vi "ADIS16470 SPI IMU.vi"() -> ()   [LabVIEW 2025]
doc: "XRS450 SPI Gyro Example\n\nThis example shows how to use the Analog Devices XRS450 gyro connected to the SPI port on the RoboRIO.\n\nThis example expects a USB cable connected from your development PC to the Type B USB Jack (next to the power input) on the roboRIO.\n\nThis example expects the Driver Station to be running."
panel:
  out "IMU Chart":T1(graph)
  in  "Calibration (sec)":dbl=4.0
  in  "Recalibrate?":bool
  out "Calibrated?":bool
  in  "Reset?":bool
  out "Device Found":bool
  in  "stop":bool
  # "Use this example to identify the X, Y, and Z axis of\nthe IMU. It also demonstrates how reset and\nrecalibration differ and lets you explore how the length\nof calibration impacts the stability of the IMU."
  # "This shows wiring for the Analog Devices ADIS16470 IMU.  It should be plugged directly into the SPI port."
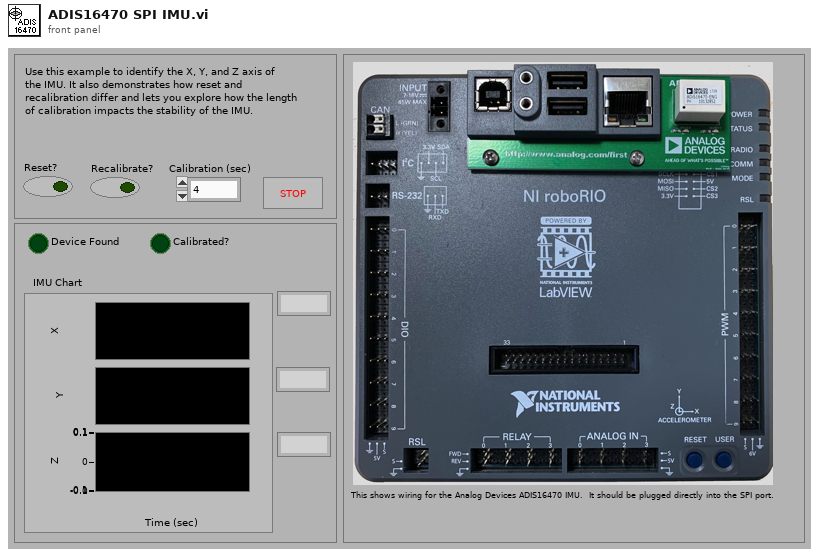
[diagram p1: front panel]
types:
  T1 = cluster{"XAngle":dbl, "YAngle":dbl, "ZAngle":dbl}
  T2 = typedef "ADIS16470 Device Reference.ctl" = cluster{"DevStatus":errorcluster, "Hardware Config":T3, "Calibration Complete":refnum<notifier>, "Status Reference":refnum<data-value>, "Data Reference":refnum<data-value>, "Sychronous Process VI":T7, "Cmd FIFO":refnum<k33>, "Source":T8, "Data FIFO":refnum<k33>, "Calibration Time (ms)":u32, "Data Reference":refnum<data-value>}
  T3 = typedef "ADIS16470 Hardware Configuration.ctl" = cluster{"SPI Clock Rate (Hz)":dbl, "IMU SPI Mode (3)":T4, "IMU Reset Pin":T5, "IMU SPI Bus":T6, "IMU Data Ready Pin":T5, "Stall Config":cluster{"Pow2BytesPerRead":u8, "StallTicks":u16, "CsToSclkTicks":u8}}
  T4 = typedef "WPI_SPIMode.ctl" = enum16{"Mode 0 (Clk Idle Low,Sample on Leading)", "Mode 1 (Clk Idle Low,Sample on Trailing)", "Mode 2 (Clk Idle High,Sample on Leading)", "Mode 3 (Clk Idle High,Sample on Trailing)"}
  T5 = typedef "FPGA_DIOChannel.ctl" = enum8{"DIO 0", "DIO 1", "DIO 2", "DIO 3", "DIO 4", "DIO 5", "DIO 6", "DIO 7", "DIO 8", "DIO 9", "DIO MXP 0", "DIO MXP 1", "DIO MXP 2", "DIO MXP 3", "DIO MXP 4", "DIO MXP 5", "DIO MXP 6", "DIO MXP 7", "DIO MXP 8", "DIO MXP 9", "DIO MXP 10", "DIO MXP 11", "DIO MXP 12", "DIO MXP 13", "DIO MXP 14", "DIO MXP 15", "SPI Port CS1", "SPI Port CS2", "SPI Port CS3", "SPI Port MISO", "SPI Port MOSI", "Invalid"}
  T6 = typedef "spi_bus.ctl" = enum16{"SPI On-Board, CS0", "SPI On-Board, CS1", "SPI On-Board, CS2", "SPI On-Board, CS3", "SPI MXP", "Invalid"}
  T7 = typedef "ADIS16470 Process.ctl" = refnum<vi>
  T8 = typedef "FPGA_CounterEncoderSourceConvertionLVSourceType.ctl" = cluster{"DevStatus":errorcluster, "AnalogTriggerMode?":bool, "DigitalMode":cluster{"DIO Channel":T9}, "AnalogTriggerMode":cluster{"AnalogTriggerIndex":T10, "OutputType":T11}}
  T9 = typedef "FPGA_DIODigitalSourceChannel.ctl" = enum8{"DIO 0", "DIO 1", "DIO 2", "DIO 3", "DIO 4", "DIO 5", "DIO 6", "DIO 7", "DIO 8", "DIO 9", "DIO MXP 0", "DIO MXP 1", "DIO MXP 2", "DIO MXP 3", "DIO MXP 4", "DIO MXP 5", "DIO MXP 6", "DIO MXP 7", "DIO MXP 8", "DIO MXP 9", "DIO MXP 10", "DIO MXP 11", "DIO MXP 12", "DIO MXP 13", "DIO MXP 14", "DIO MXP 15", "SPI Port CS1", "SPI Port CS2", "SPI Port CS3", "SPI Port MISO", "SPI Port MOSI", "Disabled"}
  T10 = typedef "FPGA_AnalogTriggerIndex.ctl" = enum8{"Trig 0", "Trig 1", "Trig 2", "Trig 3", "Trig 4", "Trig 5", "Trig 6", "Trig 7", "Invalid"}
  T11 = typedef "FPGA_AnalogTriggerOutType.ctl" = enum16{"InWindow", "TriggerState", "Rising", "Falling"}
  T12 = typedef "ADIS16470 Status.ctl" = cluster{"Calibrated?":bool, "IMU Detected?":bool}
  T13 = typedef "ADIS16470 Data.ctl" = cluster{"XAngle":dbl, "YAngle":dbl, "ZAngle":dbl}
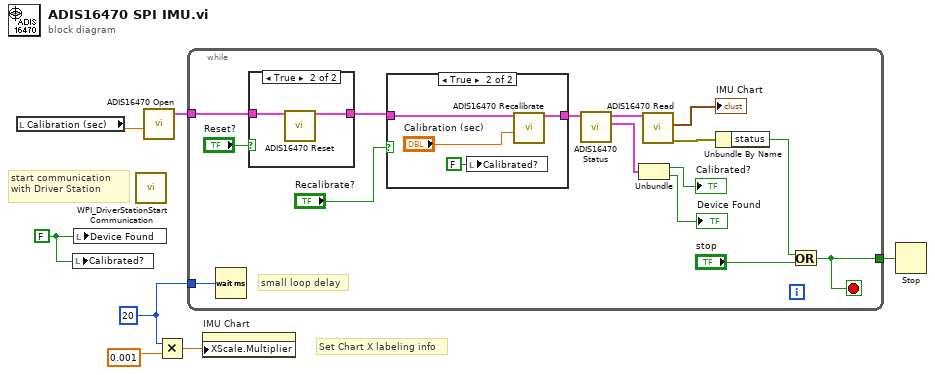
[diagram p0: block diagram]
diagram:
  w5 = u32 20 ("milliseconds to wait")
  w7 = FALSE ("Device Found")
  # "Set Chart X labeling info"
  # "start communication with Driver Station"
  n1 = local read "Calibration (sec)"() -> (w2:dbl)
  n2 = local write "Calibrated?"(w7) -> ()
  n3 = local write "Device Found"(w7) -> ()
  n4 = call <vilib>:"WPI_DriverStationStart Communication.vi"() -> ()  [unwired: 12 in]
  n5 = call <vilib>:"ADIS16470 Open.vi"("Initial Calibration Time (4s)"=w2) -> ("ADIS16470DevRef"=w1:T2)  [unwired: 9 in, 1 out]
  n6 = Multiply(x=w5, y=0.001 ("milliseconds to wait")) -> (x*y=w3:dbl)
  n7 = while {
    tunnel: w1 -> [w21]
    tunnel: [w14] -> w6
    tunnel: w5 -> [w13]
    stop <- w14 stop-if-true
    # "small loop delay"
    n8 = Wait (ms)(milliseconds to wait=w13) -> ()  [unwired: 1 out]
    n9 = case shown="True" "Reset?" {
      tunnel: w21 -> [w28 w30]
      tunnel: [w28 w29] -> w16
      frame False {
      }
      frame True {
        n10 = call <vilib>:"ADIS16470 Reset.vi"("ADIS16470DevRef"=w30) -> ("ADIS16470DevRef"=w29:T2)  [unwired: 9 in, 1 out]
      }
    }
    n11 = case shown="True" "Recalibrate?" {
      tunnel: w16 -> [w23 w26]
      tunnel: [w23 w25] -> w12
      frame False {
      }
      frame True {
        n12 = local write "Calibrated?"(FALSE ("Calibrated?")) -> ()
        n13 = call <vilib>:"ADIS16470 Recalibrate.vi"("Calibration Time (4s)"="Calibration (sec)", "ADIS16470DevRef in"=w26) -> ("ADIS16470DevRef out"=w25:T2)  [unwired: 8 in, 1 out]
      }
    }
    n14 = call <vilib>:"ADIS16470 Status.vi"("ADIS16470DevRef"=w12) -> ("ADIS16470 Status"=w11:T12, "ADIS16470DevRef"=w10:T2)  [unwired: 8 in, 1 out]
    n15 = Unbundle(w11) -> ("Calibrated?"=→"Calibrated?":bool, "IMU Detected?"=→"Device Found":bool)
    n16 = call <vilib>:"ADIS16470 Read.vi"("ADIS16470DevRef"=w10) -> ("error out"=w8:errorcluster, "ADIS16470 Value"=→"IMU Chart":T13)  [unwired: 7 in, 2 out]
    n17 = Unbundle By Name(w8) -> ("status"=w19:bool)
    n18 = Or(x=w19, y="stop") -> (x .or. y?=w14:bool)
  }
  n19 = property on="IMU Chart" class="WFChart (strict)"("XScale.Multiplier"=w3) -> ()  [unwired: 2 in, 2 out]
  n20 = Stop(stop? (T)=w6) -> ()
